vi "Package Data.vi"(8 "error in":errorcluster, 10 "DataIn":string, 11 "MC Data in":refnum<class "MC Data.lvclass">) -> (0 "error out":errorcluster, 3 "MC Data out":refnum<class "MC Data.lvclass">)   [LabVIEW 2015, in "MC Data.lvclass"]
uses:
  MC Data.lvclass
  MC Data.lvclass/MC Data.ctl
  Reusable/Data/Write measTime.vi
  Reusable/General/Atmospheric/Atmospheric Constants.vi
  Reusable/General/Atmospheric/Atmospheric Library.lvlib
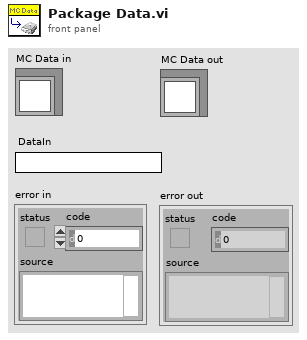
[diagram p1: front panel]
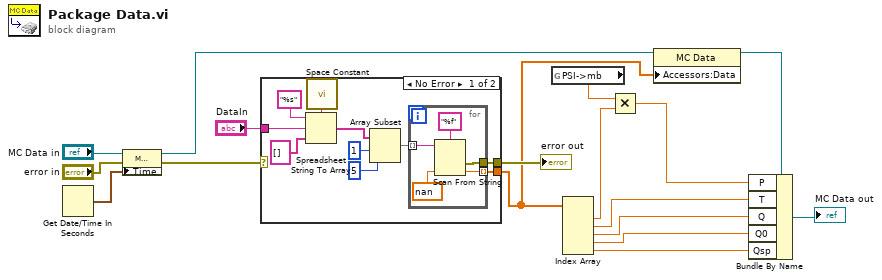
[diagram p0: block diagram]
diagram:
  n1 = Get Date/Time In Seconds() -> (seconds since 1Jan1904=w4:timestamp)
  n2 = property class="MC Data"(reference="MC Data in", error in="error in", "Time"=w4) -> (reference out=w3:refnum<class "MC Data.lvclass">, error out=w6:errorcluster)
  n3 = case shown="No Error" w6 {
    selector: w6 -> [_ w33]
    tunnel: "DataIn" -> [w24 _]
    tunnel: [w19 _] -> w1
    tunnel: [w23 w33] -> w5
    frame No Error {
      n4 = call <vilib>:"Space Constant.vi"() -> ("String"=w26:string)
      n5 = Spreadsheet String To Array(delimiter (Tab)=w26, format string="%s", spreadsheet string=w24, array type (2D Dbl)=string[] []) -> (array=w22:string[])
      n6 = Array Subset(array=w22, index=1, length=5) -> (w20:string[])
      n7 = for {
        tunnel: w20 -> [w28] mode=indexing
        tunnel: [w30] -> w19 mode=indexing
        tunnel: [w29] -> w23
        n8 = Scan From String(format string="%f", input string=w28, default 1=sgl nan ("default value 1")) -> (error out=w29:errorcluster, output 1=w30:sgl)  [unwired: 2 in, 2 out]
      }
    }
    frame Error {
    }
  }
  "error out" <- w5
  n9 = global read "Atmospheric Constants.vi" "PSI->mb"() -> (w10:sgl)
  n10 = Index Array(array=w1) -> (element #1=w15:sgl, element #2=w14:sgl, element #3=w13:sgl, element #4=w12:sgl, element #5=w11:sgl)  [unwired: 5 in]
  n11 = Multiply(x=w10, y=w15) -> (x*y=w16:sgl)
  n12 = property class="MC Data"(reference=w3, "Accessors:Data"=w1) -> (reference out=w2:refnum<class "MC Data.lvclass">)  [unwired: 1 in, 1 out]
  n13 = Bundle By Name(cluster=w2, "P"=w16, "T"=w14, "Q"=w13, "Q0"=w12, "Qsp"=w11) -> (→"MC Data out":refnum<class "MC Data.lvclass">)
